vi "Analog Inputs Updated.vi"(8 "error in":errorcluster, 10 "Analog Inputs":u16[](array[numeric]), 11 "Module ID":i32=-1) -> (0 "error out":errorcluster)   [LabVIEW 2024, in "RaspberryPiPico.lvlib"]
doc: "Analog Inputs Updated\n\n_____\nCreated using DQMH Framework: Event Scripter 7.1.0.1503."
uses:
  RaspberryPiPico.lvlib
  Analog Inputs Updated Argument--cluster.ctl
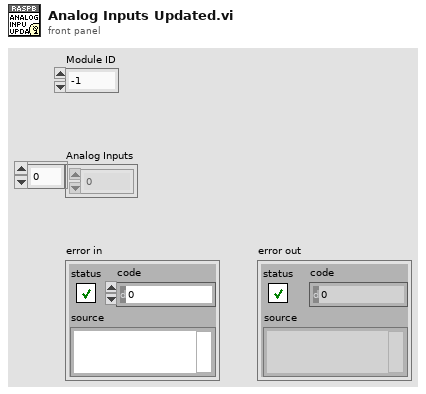
[diagram p1: front panel]
types:
  T1 = typedef "RaspberryPiPico.lvlib/Analog Inputs Updated Argument--cluster.ctl" = cluster{"Module ID":i32, "Analog Inputs":u16[]}
  T2 = typedef "RaspberryPiPico.lvlib/Broadcast Events--cluster.ctl" = cluster{"Module Did Init":refnum<user-event>, "Status Updated":refnum<user-event>, "Error Reported":refnum<user-event>, "Module Did Stop":refnum<user-event>, "Update Module Execution Status":refnum<user-event>, "Instrument Connected":refnum<user-event>, "Analog Inputs Updated":refnum<user-event>}
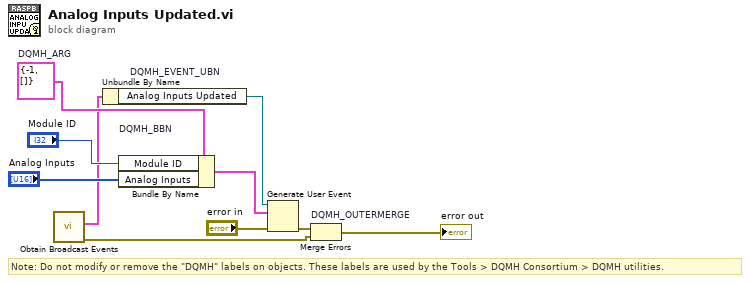
[diagram p0: block diagram]
diagram:
  w5 = T1 {"Module ID"=-1, "Analog Inputs"=[]}  # DQMH_ARG
  # "Note: Do not modify or remove the \"DQMH\" labels on objects. These labels are used by the Tools > DQMH Consortium > DQMH utilities."
  n1 = call "Obtain Broadcast Events.vi"() -> ("error out"=w2:errorcluster, "RaspberryPiPico Broadcast Events"=w1:T2)  [unwired: 10 in]
  n2 = Unbundle By Name "DQMH_EVENT_UBN"(w1) -> ("Analog Inputs Updated"=w7:refnum<user-event>)
  n3 = Bundle By Name "DQMH_BBN"(cluster=w5, "Module ID"="Module ID", "Analog Inputs"="Analog Inputs") -> (w8:T1)
  n4 = Generate User Event(user event=w7, event data cluster=w8, error in="error in") -> (error out=w6:errorcluster)  [unwired: 1 in, 1 out]
  n5 = Merge Errors "DQMH_OUTERMERGE"(w6, w2) -> (→"error out":errorcluster)
